vi "negative2scomplement_to_integer.vi"(11 "BYTE":u8) -> (3 "Result":u8)   [LabVIEW 2012]
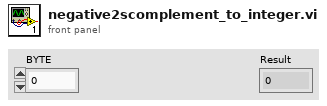
[diagram p1: front panel]
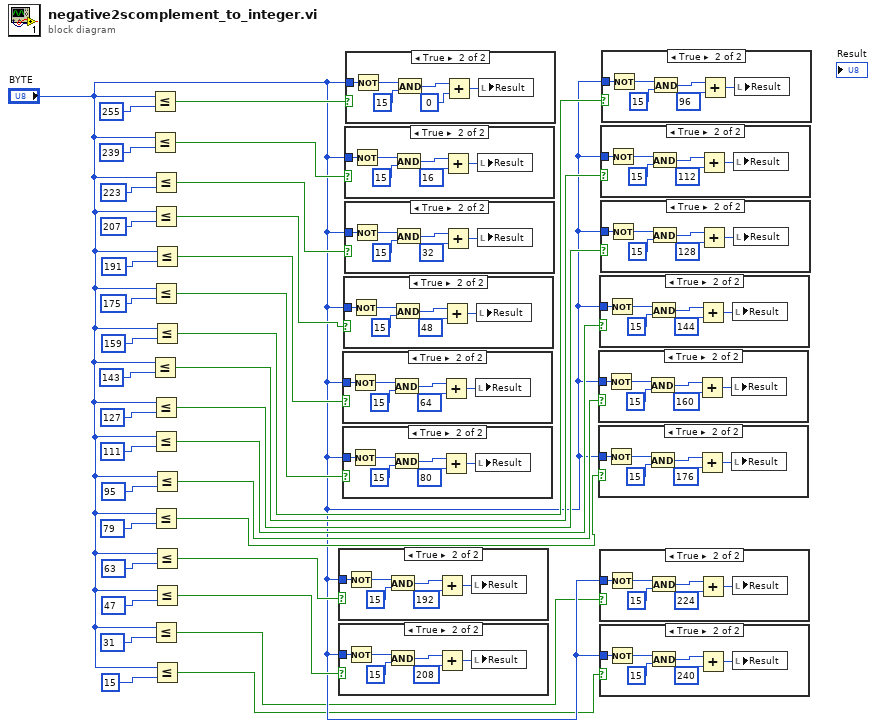
[diagram p0: block diagram]
diagram:
  n1 = Less Or Equal?(x="BYTE", y=u8 255) -> (x <= y?=w17:bool)
  n2 = Less Or Equal?(x="BYTE", y=u8 239) -> (x <= y?=w16:bool)
  n3 = Less Or Equal?(x="BYTE", y=u8 143) -> (x <= y?=w10:bool)
  n4 = Less Or Equal?(x="BYTE", y=u8 223) -> (x <= y?=w15:bool)
  n5 = Less Or Equal?(x="BYTE", y=u8 207) -> (x <= y?=w14:bool)
  n6 = Less Or Equal?(x="BYTE", y=u8 175) -> (x <= y?=w12:bool)
  n7 = Less Or Equal?(x="BYTE", y=u8 127) -> (x <= y?=w9:bool)
  n8 = Less Or Equal?(x="BYTE", y=u8 111) -> (x <= y?=w8:bool)
  n9 = Less Or Equal?(x="BYTE", y=u8 79) -> (x <= y?=w6:bool)
  n10 = Less Or Equal?(x="BYTE", y=u8 31) -> (x <= y?=w2:bool)
  n11 = Less Or Equal?(x="BYTE", y=u8 191) -> (x <= y?=w13:bool)
  n12 = Less Or Equal?(x="BYTE", y=u8 159) -> (x <= y?=w11:bool)
  n13 = Less Or Equal?(x="BYTE", y=u8 95) -> (x <= y?=w7:bool)
  n14 = Less Or Equal?(x="BYTE", y=u8 63) -> (x <= y?=w5:bool)
  n15 = Less Or Equal?(x="BYTE", y=u8 47) -> (x <= y?=w4:bool)
  n16 = Less Or Equal?(x="BYTE", y=u8 15) -> (x <= y?=w1:bool)
  n17 = case shown="True" w5 {
    tunnel: "BYTE" -> [_ w35]
    frame False {
    }
    frame True {
      n18 = Not(x=w35) -> (.not. x?=w36:u8)
      n19 = And(x=w36, y=u8 15) -> (x .and. y?=w38:u8)
      n20 = Add(x=w38, y=u8 192) -> (x+y=w34:u8)
      n21 = local write "Result"(w34) -> ()
    }
  }
  n22 = case shown="True" w4 {
    tunnel: "BYTE" -> [_ w41]
    frame False {
    }
    frame True {
      n23 = Not(x=w41) -> (.not. x?=w42:u8)
      n24 = And(x=w42, y=u8 15) -> (x .and. y?=w44:u8)
      n25 = Add(x=w44, y=u8 208) -> (x+y=w40:u8)
      n26 = local write "Result"(w40) -> ()
    }
  }
  n27 = case shown="True" w13 {
    tunnel: "BYTE" -> [_ w47]
    frame False {
    }
    frame True {
      n28 = Not(x=w47) -> (.not. x?=w48:u8)
      n29 = And(x=w48, y=u8 15) -> (x .and. y?=w50:u8)
      n30 = Add(x=w50, y=u8 64) -> (x+y=w46:u8)
      n31 = local write "Result"(w46) -> ()
    }
  }
  n32 = case shown="True" w12 {
    tunnel: "BYTE" -> [_ w53]
    frame False {
    }
    frame True {
      n33 = Not(x=w53) -> (.not. x?=w54:u8)
      n34 = And(x=w54, y=u8 15) -> (x .and. y?=w56:u8)
      n35 = Add(x=w56, y=u8 80) -> (x+y=w52:u8)
      n36 = local write "Result"(w52) -> ()
    }
  }
  n37 = case shown="True" w14 {
    tunnel: "BYTE" -> [_ w59]
    frame False {
    }
    frame True {
      n38 = Not(x=w59) -> (.not. x?=w60:u8)
      n39 = And(x=w60, y=u8 15) -> (x .and. y?=w62:u8)
      n40 = Add(x=w62, y=u8 48) -> (x+y=w58:u8)
      n41 = local write "Result"(w58) -> ()
    }
  }
  n42 = case shown="True" w16 {
    tunnel: "BYTE" -> [_ w65]
    frame False {
    }
    frame True {
      n43 = Not(x=w65) -> (.not. x?=w66:u8)
      n44 = And(x=w66, y=u8 15) -> (x .and. y?=w68:u8)
      n45 = Add(x=w68, y=u8 16) -> (x+y=w64:u8)
      n46 = local write "Result"(w64) -> ()
    }
  }
  n47 = case shown="True" w15 {
    tunnel: "BYTE" -> [_ w71]
    frame False {
    }
    frame True {
      n48 = Not(x=w71) -> (.not. x?=w72:u8)
      n49 = And(x=w72, y=u8 15) -> (x .and. y?=w74:u8)
      n50 = Add(x=w74, y=u8 32) -> (x+y=w70:u8)
      n51 = local write "Result"(w70) -> ()
    }
  }
  n52 = case shown="True" w17 {
    tunnel: "BYTE" -> [_ w77]
    frame False {
    }
    frame True {
      n53 = Not(x=w77) -> (.not. x?=w78:u8)
      n54 = And(x=w78, y=u8 15) -> (x .and. y?=w80:u8)
      n55 = Add(x=w80, y=u8 0) -> (x+y=w76:u8)
      n56 = local write "Result"(w76) -> ()
    }
  }
  n57 = case shown="True" w7 {
    tunnel: "BYTE" -> [_ w83]
    frame False {
    }
    frame True {
      n58 = Not(x=w83) -> (.not. x?=w84:u8)
      n59 = And(x=w84, y=u8 15) -> (x .and. y?=w86:u8)
      n60 = Add(x=w86, y=u8 160) -> (x+y=w82:u8)
      n61 = local write "Result"(w82) -> ()
    }
  }
  n62 = case shown="True" w6 {
    tunnel: "BYTE" -> [_ w89]
    frame False {
    }
    frame True {
      n63 = Not(x=w89) -> (.not. x?=w90:u8)
      n64 = And(x=w90, y=u8 15) -> (x .and. y?=w92:u8)
      n65 = Add(x=w92, y=u8 176) -> (x+y=w88:u8)
      n66 = local write "Result"(w88) -> ()
    }
  }
  n67 = case shown="True" w8 {
    tunnel: "BYTE" -> [_ w95]
    frame False {
    }
    frame True {
      n68 = Not(x=w95) -> (.not. x?=w96:u8)
      n69 = And(x=w96, y=u8 15) -> (x .and. y?=w98:u8)
      n70 = Add(x=w98, y=u8 144) -> (x+y=w94:u8)
      n71 = local write "Result"(w94) -> ()
    }
  }
  n72 = case shown="True" w2 {
    tunnel: "BYTE" -> [_ w101]
    frame False {
    }
    frame True {
      n73 = Not(x=w101) -> (.not. x?=w102:u8)
      n74 = And(x=w102, y=u8 15) -> (x .and. y?=w104:u8)
      n75 = Add(x=w104, y=u8 224) -> (x+y=w100:u8)
      n76 = local write "Result"(w100) -> ()
    }
  }
  n77 = case shown="True" w1 {
    tunnel: "BYTE" -> [_ w107]
    frame False {
    }
    frame True {
      n78 = Not(x=w107) -> (.not. x?=w108:u8)
      n79 = And(x=w108, y=u8 15) -> (x .and. y?=w110:u8)
      n80 = Add(x=w110, y=u8 240) -> (x+y=w106:u8)
      n81 = local write "Result"(w106) -> ()
    }
  }
  n82 = case shown="True" w10 {
    tunnel: "BYTE" -> [_ w113]
    frame False {
    }
    frame True {
      n83 = Not(x=w113) -> (.not. x?=w114:u8)
      n84 = And(x=w114, y=u8 15) -> (x .and. y?=w116:u8)
      n85 = Add(x=w116, y=u8 112) -> (x+y=w112:u8)
      n86 = local write "Result"(w112) -> ()
    }
  }
  n87 = case shown="True" w9 {
    tunnel: "BYTE" -> [_ w119]
    frame False {
    }
    frame True {
      n88 = Not(x=w119) -> (.not. x?=w120:u8)
      n89 = And(x=w120, y=u8 15) -> (x .and. y?=w122:u8)
      n90 = Add(x=w122, y=u8 128) -> (x+y=w118:u8)
      n91 = local write "Result"(w118) -> ()
    }
  }
  n92 = case shown="True" w11 {
    tunnel: "BYTE" -> [_ w125]
    frame False {
    }
    frame True {
      n93 = Not(x=w125) -> (.not. x?=w126:u8)
      n94 = And(x=w126, y=u8 15) -> (x .and. y?=w128:u8)
      n95 = Add(x=w128, y=u8 96) -> (x+y=w124:u8)
      n96 = local write "Result"(w124) -> ()
    }
  }
